vi "Sxx Measurements to Capacitance.vi"(7 "Sweep Frequency Start":dbl, 8 "error in (no error)":errorcluster, 11 "S11 Data":cdb[](array[numeric])) -> (0 "error out":errorcluster, 3 "Capacitance":dbl[](array[numeric]))   [LabVIEW 2013]
doc: "Converts the raw S11 data from niVNA fetch into capacitance measurement."
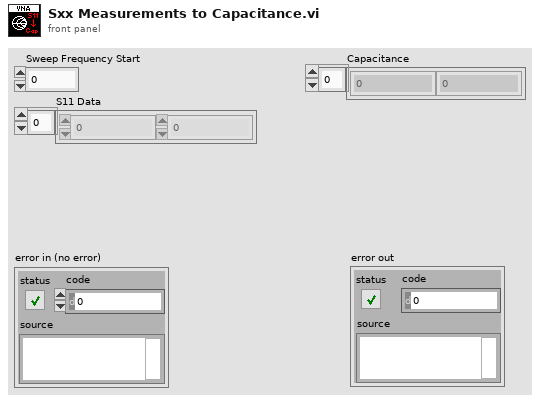
[diagram p1: front panel]
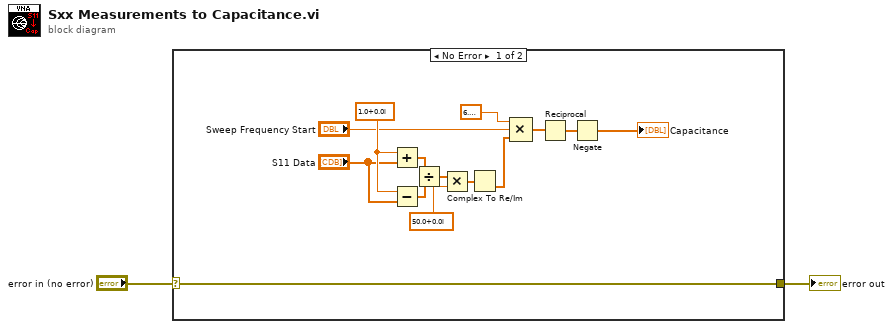
[diagram p0: block diagram]
diagram:
  n1 = case shown="No Error" "error in (no error)" {
    selector: "error in (no error)" -> [w3 w17]
    tunnel: [w3 w17] -> w2
    frame No Error {
      w16 = cdb 1.0+0.0i
      n2 = Add(x=w16, y="S11 Data") -> (x+y=w15:cdb[])
      n3 = Subtract(x=w16, y="S11 Data") -> (x-y=w14:cdb[])
      n4 = Divide(x=w15, y=w14) -> (x/y=w13:cdb[])
      n5 = Multiply(x=w13, y=cdb 50.0+0.0i) -> (x*y=w11:cdb[])
      n6 = Complex To Re/Im(x + iy=w11) -> (y=w7:dbl[])  [unwired: 1 out]
      n7 = Compound Arithmetic op=MULTIPLY(6.283185307179586, "Sweep Frequency Start", w7) -> (w9:dbl[])
      n8 = Reciprocal(x=w9) -> (1/x=w8:dbl[])
      n9 = Negate(x=w8) -> (-x=→"Capacitance":dbl[])
    }
    frame Error {
    }
  }
  "error out" <- w2
